vi "OrderExecuted.vi"(11 "buffer.in":u64[](array[numeric])=[0, 0, 0, 0, 0, 0, 0, 0, 0] format="%.0x") -> (3 "OrderBook.Command":T1)   [LabVIEW 2020]
uses:
  Market.Data.Common/fpga/orderbook.command.ctl
  Market.Data.Common/fpga/orderbook.command.type.ctl
  Market.Data.Common/fpga/fpganow.common.fpga.lvlib
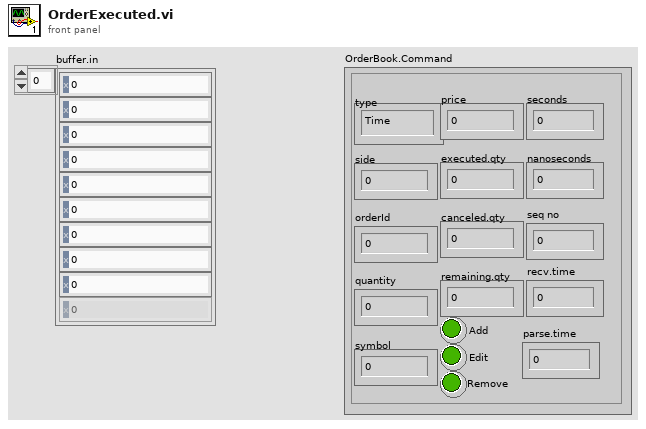
[diagram p1: front panel]
types:
  T1 = typedef "fpganow.common.fpga.lvlib/orderbook.command.ctl" = cluster{"type":T2, "side":u8, "orderId ":u64, "quantity":u32, "symbol":u64, "price":u64, "executed.qty":u32, "canceled.qty":u32, "remaining.qty":u32, "seconds":u64, "nanoseconds":u64, "Add":bool, "Edit":bool, "Remove":bool, "seq no":u32, "recv.time":u64, "parse.time":u64}
  T2 = typedef "fpganow.common.fpga.lvlib/orderbook.command.type.ctl" = enum8{"Time", "AddOrder", "OrderExecuted", "OrderExecutedAtPrice", "ReduceSize", "ModifyOrder", "DeleteOrder", "Get.Everything", "Get.All.Orders", "Get.Top"}
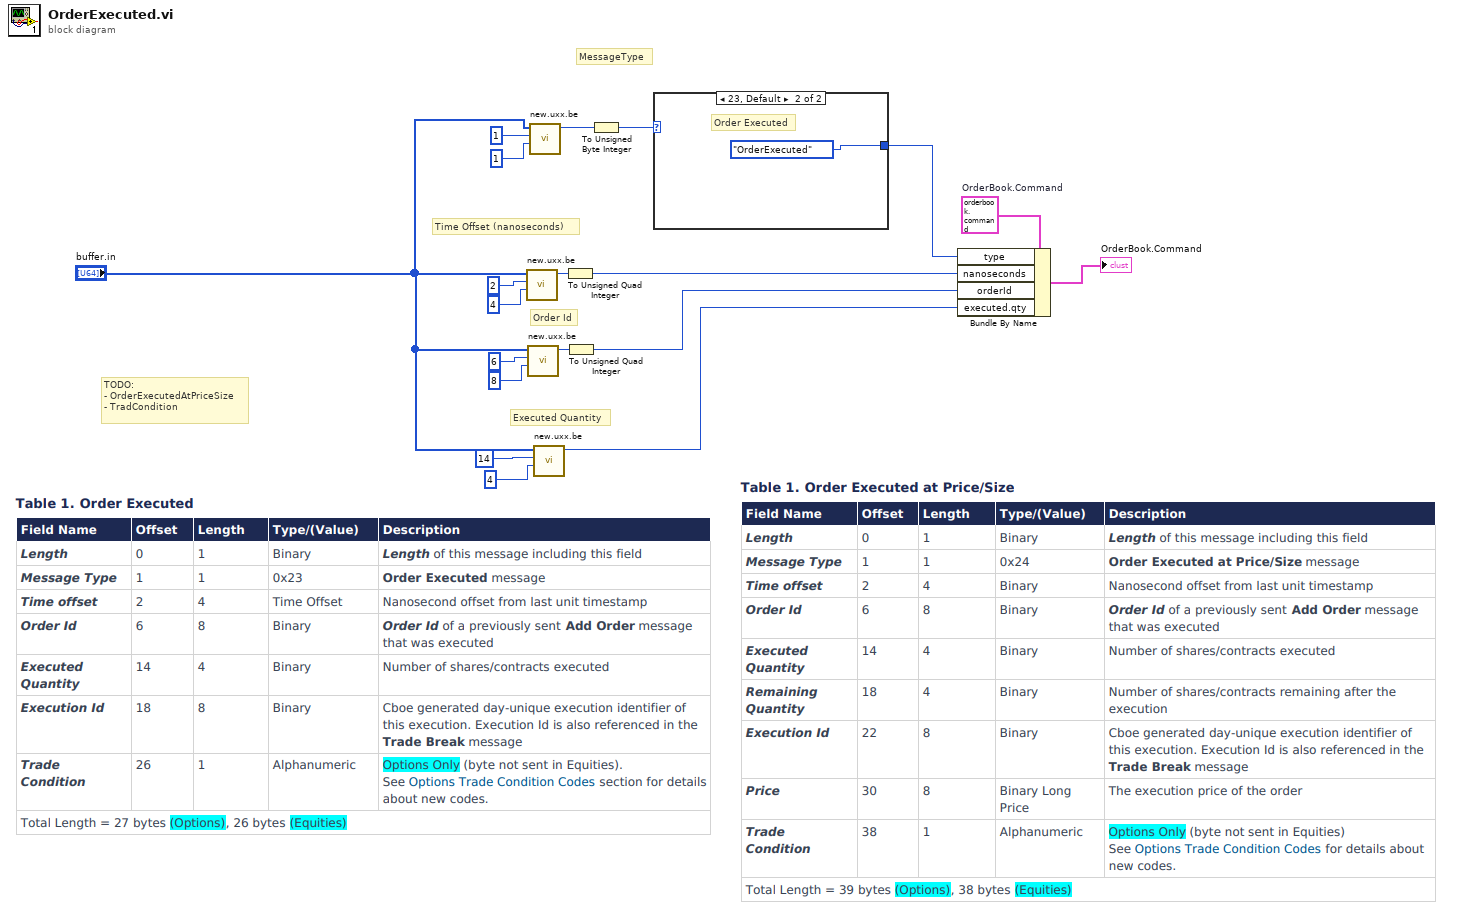
[diagram p0: block diagram]
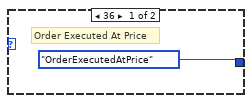
[diagram p2: hidden frame]
diagram:
  w15 = T1 {"type"=enum."AddOrder", "side"=0, "orderId "=0, "quantity"=0, "symbol"=0, "price"=0, "executed.qty"=0, "canceled.qty"=0, "remaining.qty"=0, "seconds"=0, "nanoseconds"=0, "Add"=FALSE, "Edit"=FALSE, "Remove"=FALSE, "seq no"=0, "recv.time"=0, "parse.time"=0}  # OrderBook.Command
  # "MessageType"
  # "TODO:\n- OrderExecutedAtPriceSize\n- TradCondition"
  # "Executed Quantity"
  # "Order Id"
  # "Time Offset (nanoseconds)"
  n1 = call "new.uxx.be.vi"("buffer (U64)"="buffer.in", "Start.Idx"=u8 2, "Length"=u8 4) -> ("Out.Value U64"=w16:u64)  [unwired: 7 in]
  n2 = call "new.uxx.be.vi"("buffer (U64)"="buffer.in", "Start.Idx"=u8 6, "Length"=u8 8) -> ("Out.Value U64"=w11:u64)  [unwired: 7 in]
  n3 = call "new.uxx.be.vi"("buffer (U64)"="buffer.in", "Start.Idx"=u8 1, "Length"=u8 1) -> ("Out.Value U64"=w4:u64)  [unwired: 7 in]
  n4 = call "new.uxx.be.vi"("buffer (U64)"="buffer.in", "Start.Idx"=u8 14, "Length"=u8 4 ("Start.Idx")) -> ("Out.Value U64"=w9:u64)  [unwired: 7 in]
  n5 = To Unsigned Quad Integer(1:w16) -> (0:w19:u64)
  n6 = To Unsigned Quad Integer(1:w11) -> (0:w10:u64)
  n7 = To Unsigned Byte Integer(number=w4) -> (unsigned 8bit integer=w2:u8)
  n8 = case shown="23, Default" w2 {
    tunnel: [orderbook.command.type."OrderExecutedAtPrice" ("OrderBook Command") orderbook.command.type."OrderExecuted" ("OrderBook Command")] -> w1
    frame 36 {
      # "Order Executed At Price"
    }
    frame 35, Default {
      # "Order Executed"
    }
  }
  n9 = Bundle By Name(cluster=w15, "type"=w1, "nanoseconds"=w19, "orderId"=w10, "executed.qty"=w9) -> (→"OrderBook.Command":T1)
